vi "Runtime Test.vi"() -> ()   [LabVIEW 2017, in "ThreePhasePLL tests.lvlib"]
uses:
  ThreePhasePLL tests.lvlib
  module/execution/ThreePhasePLL runtime.lvclass
  <vilib>/NI/Tag Bus/dictionary/data dictionary.lvclass/data dictionary.ctl
  <vilib>/NI/Tag Bus/dictionary/lookup polymorphs/locate double.vi
  <vilib>/NI/Tag Bus/table/data polymorphs/read one/read Double.vi
  <vilib>/NI/Tag Bus/table/data polymorphs/write one/write Double.vi
  <vilib>/NI/Tag Bus/dictionary/search/find data index.vi
  <vilib>/NI/Tag Bus/dictionary/search/search string list.vi
  module/configuration/ThreePhasePLL configuration.lvclass
  C:/Program Files (x86)/National Instruments/LabVIEW 2017/vi.lib/NI/Tag Bus Module Framework/module configuration/TBM module configuration.lvclass
  <vilib>/NI/Tag Bus/dictionary/tag not found.vi
  <vilib>/NI/Tag Bus/dictionary/data dictionary.lvclass
  <vilib>/NI/Tag Bus/table/data table.lvlib
panel:
  out "input lookup error":errorcluster
  out "input error":errorcluster
  out "process result lookup error":errorcluster
  out "final error":errorcluster
  out "output error":errorcluster
  out "process error":errorcluster
  out "output lookup error":errorcluster
  out "process parameter  lookup error":errorcluster
  out "correct execution settings":bool
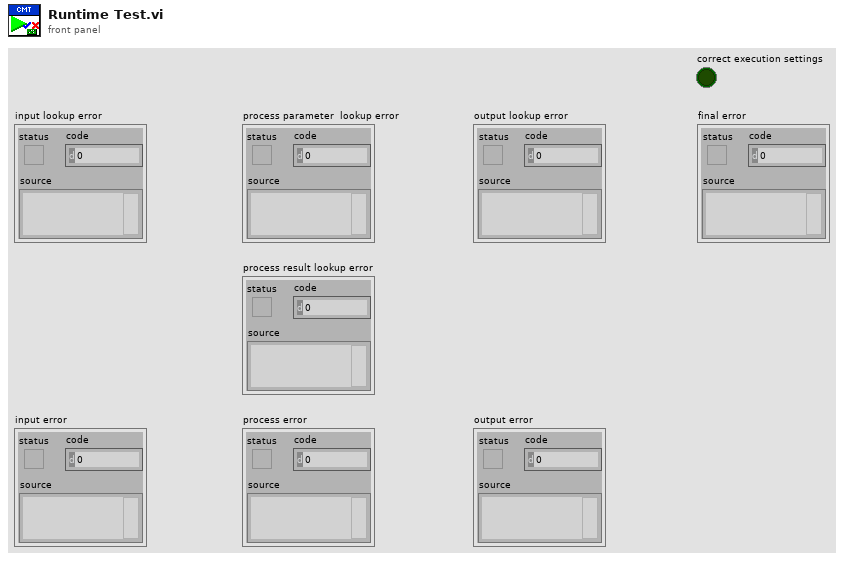
[diagram p1: front panel]
types:
  T1 = typedef "TBM channel.lvclass/data tables.ctl" = cluster{"input data":T2, "processing parameter":T2, "processing result":T2, "output data":T2}
  T2 = typedef "tag bus.lvlib/dictionary table pair.ctl" = cluster{"data dictionary":refnum<class "data dictionary.lvclass">, "data table":T3}
  T3 = typedef "tag bus.lvlib/data table.lvlib/data table.ctl" = cluster{"Double":dbl[], "Single":sgl[], "I64":i64[], "I32":i32[], "I16":i16[], "I8":i8[], "U64":u64[], "U32":u32[], "U16":u16[], "U8":u8[], "Boolean":bool[], "String":string[], "Array of Double":cluster{"DBL Array":dbl[]}[], "Array of Single":cluster{"SGL Array":sgl[]}[], "Array of I64":cluster{"I64 Array":i64[]}[], "Array of I32":cluster{"I32 Array":i32[]}[], "Array of I16":cluster{"I16 Array":i16[]}[], "Array of I8":cluster{"I8 Array":i8[]}[], "Array of U64":cluster{"U64 Array":u64[]}[], "Array of U32":cluster{"U32 Array":u32[]}[], "Array of U16":cluster{"U16 Array":u16[]}[], "Array of U8":cluster{"U8 Array":u8[]}[], "Array of Boolean":cluster{"Boolean Array":bool[]}[], "Array of String":cluster{"String Array":string[]}[]}
  T4 = typedef "TBM module execution interface.lvclass/execution settings.ctl" = cluster{"reads inputs":bool, "processes data":bool, "writes outputs":bool}
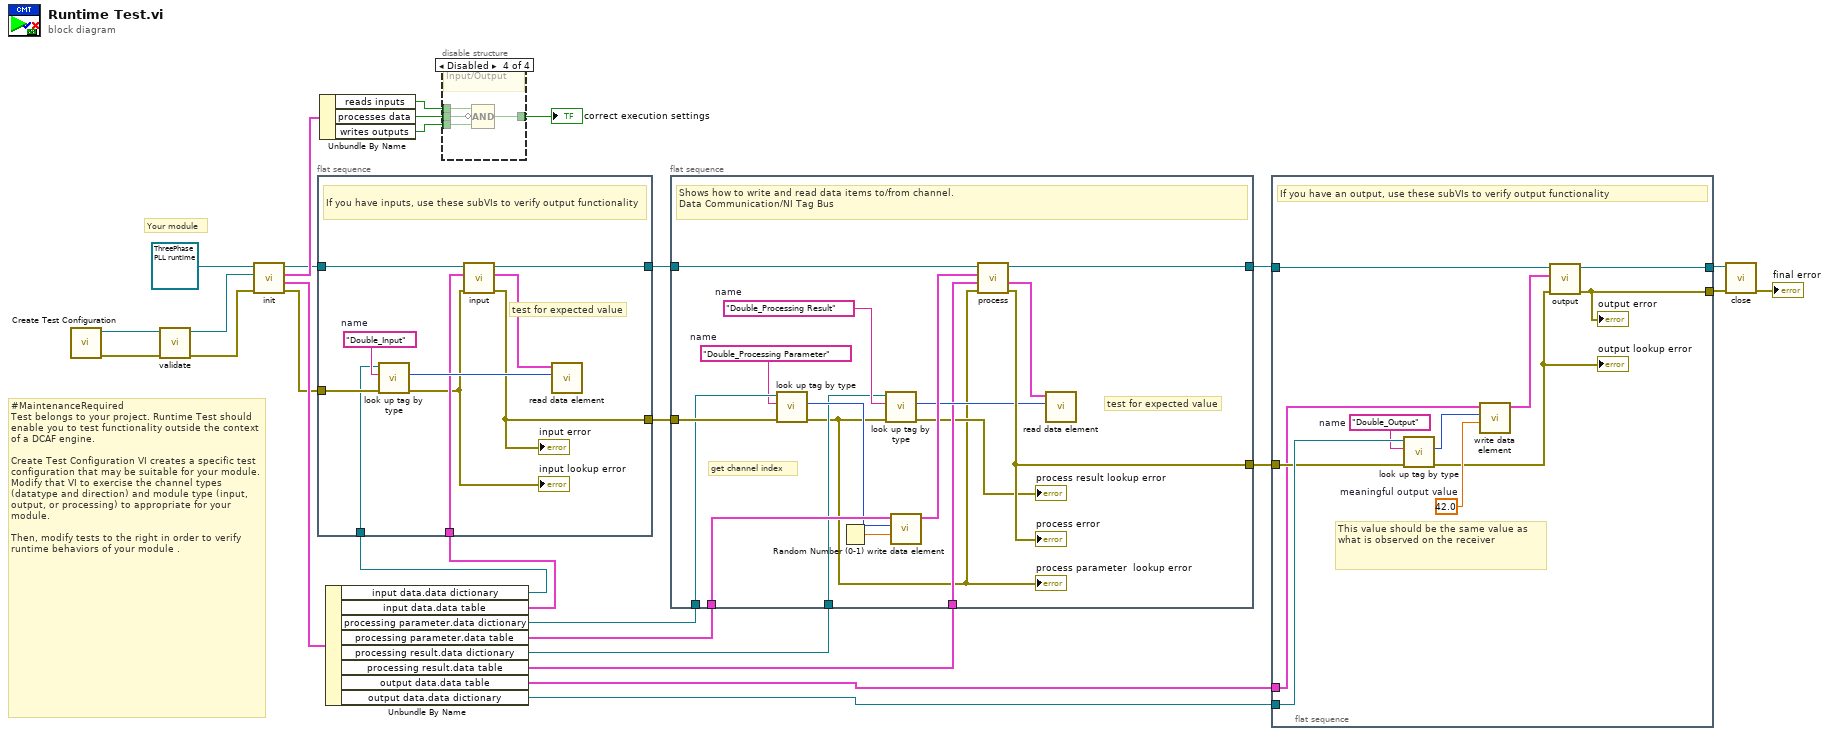
[diagram p0: block diagram]
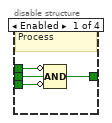
[diagram p2: hidden frame]
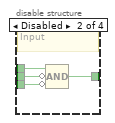
[diagram p3: hidden frame]
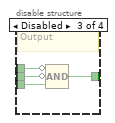
[diagram p4: hidden frame]
diagram:
  # "Your module"
  # "#MaintenanceRequired\nTest belongs to your project. Runtime Test should enable you to test functionality outside the context of a DCAF engine. \n\nCreate Test Configuration VI creates a specific test configuration that may be suitable for your module. Modify that VI to exercise the channel types (datatype and direction) and module type (input, output, or processing) to appropriate for your module. \n\nThen, modify tests to the right in order to verify runtime behaviors of your module ."
  n1 = call "Create Test Configuration.vi"() -> ("error out"=w9:errorcluster, "Module"=w11:refnum<class "ThreePhasePLL configuration.lvclass">)  [unwired: 6 in, 4 out]
  n2 = call-dynamic "validate.vi"("error in"=w9, "fixed channel configuration in"=w11) -> ("error out"=w27:errorcluster, "fixed channel configuration out"=w28:refnum<class "ThreePhasePLL configuration.lvclass">)  [unwired: 8 in]
  n3 = call-dynamic "init.vi"("error in"=w27, "TBM module configuration in"=w28, "fixed channel runtime in"=refnum<class "ThreePhasePLL runtime.lvclass"> refnum ("user module")) -> ("error out"=w8:errorcluster, "data allocations"=w22:T1, "execution settings"=w26:T4, "fixed channel runtime out"=w6:refnum<class "ThreePhasePLL runtime.lvclass">)  [unwired: 5 in]
  n4 = flat-sequence {
    tunnel: w8 -> [w35]
    tunnel: [w30] -> w7
    tunnel: w6 -> [w38]
    tunnel: [w37] -> w5
    tunnel: w4 -> [w34]
    tunnel: w1 -> [w31]
    frame #0 {
      w36 = "Double_Input"  # name
      # "test for expected value"
      # "If you have inputs, use these subVIs to verify output functionality"
      n5 = call-poly <vilib>:"look up tag by type.vi"("error in"=w35, "name"=w36, "data dictionary in"=w34) -> ("error out"=w29:errorcluster, "index"=w32:i32)  [unwired: 6 in, 1 out]
      "input lookup error" <- w29
      n6 = call-dynamic "input.vi"("error in"=w29, "input allocation"=w31, "ThreePhasePLL runtime in"=w38) -> ("error out"=w30:errorcluster, "input data"=w33:T3, "ThreePhasePLL runtime out"=w37:refnum<class "ThreePhasePLL runtime.lvclass">)  [unwired: 6 in]
      "input error" <- w30
      n7 = call-poly <vilib>:"read data element.vi"("index"=w32, "data table in"=w33) -> ()  [unwired: 8 in, 2 out]
    }
  }
  n8 = Unbundle By Name(w26) -> ("reads inputs"=w24:bool, "processes data"=w12:bool, "writes outputs"=w25:bool)
  n9 = Unbundle By Name(w22) -> ("input data.data dictionary"=w4:refnum<class "data dictionary.lvclass">, "input data.data table"=w1:T3, "processing parameter.data dictionary"=w21:refnum<class "data dictionary.lvclass">, "processing parameter.data table"=w20:T3, "processing result.data dictionary"=w3:refnum<class "data dictionary.lvclass">, "processing result.data table"=w2:T3, "output data.data table"=w13:T3, "output data.data dictionary"=w19:refnum<class "data dictionary.lvclass">)
  n10 = disable-structure shown="Disabled" {
    disable-tunnel: w25 -> [w42 w46 w50 w54]
    disable-tunnel: w24 -> [w41 w45 w49 w53]
    disable-tunnel: [w40 w44 w48 w52] -> w23
    disable-tunnel: w12 -> [w39 w43 w47 w51]
    frame Enabled {
      # "Process"
      n11 = Compound Arithmetic op=AND(invert w41, w39, invert w42) -> (w40:bool)
    }
    frame Disabled {
      # "Input"
      n12 = Compound Arithmetic op=AND(w45, invert w43, invert w46) -> (w44:bool)
    }
    frame Disabled {
      # "Output"
      n13 = Compound Arithmetic op=AND(invert w49, invert w47, w50) -> (w48:bool)
    }
    frame Disabled {
      # "Input/Output"
      n14 = Compound Arithmetic op=AND(w53, invert w51, w54) -> (w52:bool)
    }
  }
  "correct execution settings" <- w23
  n15 = flat-sequence {
    tunnel: w21 -> [w61]
    tunnel: w7 -> [w62]
    tunnel: w20 -> [w71]
    tunnel: [w70] -> w15
    tunnel: [w69] -> w14
    tunnel: w5 -> [w66]
    tunnel: w3 -> [w59]
    tunnel: w2 -> [w57]
    frame #0 {
      w60 = "Double_Processing Parameter"  # name
      w64 = "Double_Processing Result"  # name
      # "test for expected value"
      # "get channel index"
      # "Shows how to write and read data items to/from channel.\nData Communication/NI Tag Bus"
      n16 = call-poly <vilib>:"look up tag by type.vi"("error in"=w62, "name"=w60, "data dictionary in"=w61) -> ("error out"=w55:errorcluster, "index"=w63:i32)  [unwired: 6 in, 1 out]
      "process parameter  lookup error" <- w55
      n17 = Random Number (0-1)() -> (number: 0 to 1=w67:dbl)
      n18 = call-poly <vilib>:"look up tag by type.vi"("error in"=w55, "name"=w64, "data dictionary in"=w59) -> ("error out"=→"process result lookup error":errorcluster, "index"=w65:i32)  [unwired: 6 in, 1 out]
      n19 = call-poly <vilib>:"write data element.vi"("value"=w67, "index"=w63, "data table in"=w71) -> ("data table out"=w68:T3)  [unwired: 8 in]
      n20 = call-dynamic "process.vi"("error in"=w55, "result allocation"=w57, "parameters"=w68, "ThreePhasePLL runtime in"=w66) -> ("error out"=w69:errorcluster, "results"=w58:T3, "ThreePhasePLL runtime out"=w70:refnum<class "ThreePhasePLL runtime.lvclass">)  [unwired: 4 in, 1 out]
      "process error" <- w69
      n21 = call-poly <vilib>:"read data element.vi"("index"=w65, "data table in"=w58) -> ()  [unwired: 8 in, 2 out]
    }
  }
  n22 = flat-sequence {
    tunnel: w19 -> [w82]
    tunnel: [w78] -> w18
    tunnel: [w77] -> w17
    tunnel: w15 -> [w76]
    tunnel: w14 -> [w75]
    tunnel: w13 -> [w74]
    frame #0 {
      w72 = "Double_Output"  # name
      w80 = 42.0  # meaningful output value
      # "This value should be the same value as what is observed on the receiver"
      # "If you have an output, use these subVIs to verify output functionality"
      n23 = call-poly <vilib>:"look up tag by type.vi"("error in"=w75, "name"=w72, "data dictionary in"=w82) -> ("error out"=w73:errorcluster, "index"=w81:i32)  [unwired: 6 in, 1 out]
      "output lookup error" <- w73
      n24 = call-poly <vilib>:"write data element.vi"("value"=w80, "index"=w81, "data table in"=w74) -> ("data table out"=w79:T3)  [unwired: 8 in]
      n25 = call-dynamic "output.vi"("error in"=w73, "output data"=w79, "ThreePhasePLL runtime in"=w76) -> ("error out"=w77:errorcluster, "ThreePhasePLL runtime out"=w78:refnum<class "ThreePhasePLL runtime.lvclass">)  [unwired: 6 in, 1 out]
      "output error" <- w77
    }
  }
  n26 = call-dynamic "close.vi"("error in"=w17, "module in"=w18) -> ("error out"=→"final error":errorcluster)  [unwired: 9 in]
